vi "FOD.vi"(7 "Yaw":dbl, 8 "DriveMode":enum16{"Meccanum", "Traction"}(ring), 9 "Rotation in":dbl, 10 "Y in":dbl, 11 "X in":dbl) -> (1 "Rotation out":dbl, 2 "Y out":dbl, 3 "X out":dbl)   [LabVIEW 2013]
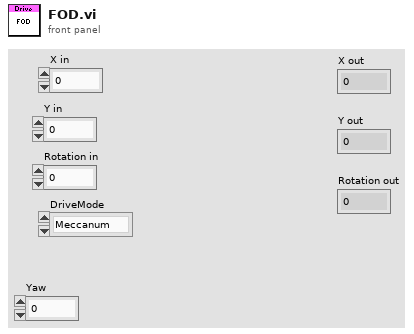
[diagram p1: front panel]
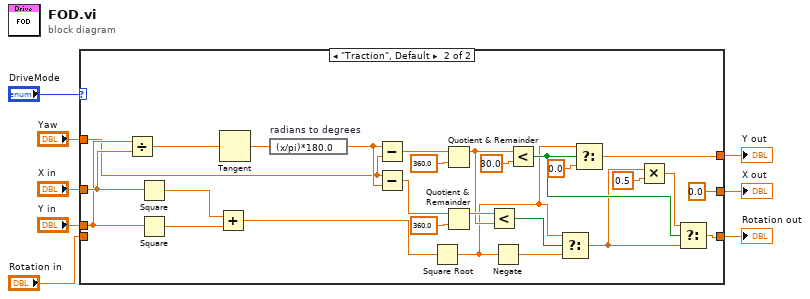
[diagram p0: block diagram]
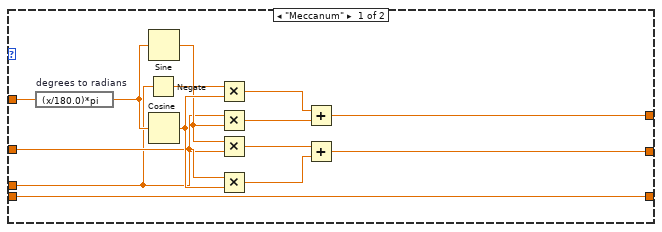
[diagram p2: hidden frame]
diagram:
  n1 = case shown="\"Traction\", Default" "DriveMode" {
    tunnel: [w13 0.0] -> w6
    tunnel: [w14 w38] -> w7
    tunnel: [w12 w35] -> w5
    tunnel: "Rotation in" -> [w12 _]
    tunnel: "X in" -> [w11 w40]
    tunnel: "Y in" -> [w10 w39]
    tunnel: "Yaw" -> [w9 w23]
    frame "Meccanum" {
      n2 = expression code="(x/180.0)*pi" "degrees to radians"(w9) -> (w18:dbl)
      n3 = Negate(x=w10) -> (-x=w15:dbl)
      n4 = Sine(x=w18) -> (sin(x)=w19:dbl)
      n5 = Cosine(x=w18) -> (cos(x)=w20:dbl)
      n6 = Multiply(x=w15, y=w20) -> (x*y=w16:dbl)
      n7 = Multiply(x=w11, y=w19) -> (x*y=w17:dbl)
      n8 = Multiply(x=w19, y=w10) -> (x*y=w21:dbl)
      n9 = Multiply(x=w11, y=w20) -> (x*y=w22:dbl)
      n10 = Add(x=w16, y=w17) -> (x+y=w14:dbl)
      n11 = Add(x=w21, y=w22) -> (x+y=w13:dbl)
    }
    frame "Traction", Default {
      n12 = Divide(x=w39, y=w40) -> (x/y=w49:dbl)
      n13 = Square(x=w40) -> (x^2=w41:dbl)
      n14 = Square(x=w39) -> (x^2=w42:dbl)
      n15 = Add(x=w41, y=w42) -> (x+y=w43:dbl)
      n16 = Tangent(1:w49) -> (0:w48:dbl)
      n17 = expression code="(x/pi)*180.0" "radians to degrees"(w48) -> (w32:dbl)
      n18 = Subtract(x=w32, y=w23) -> (x-y=w46:dbl)
      n19 = Subtract(x=w23, y=w32) -> (x-y=w33:dbl)
      n20 = Square Root(x=w43) -> (sqrt(x)=w24:dbl)
      n21 = Quotient & Remainder(x=w46, y=360.0) -> (x-y*floor(x/y)=w30:dbl)  [unwired: 1 out]
      n22 = Quotient & Remainder(x=w33, y=360.0) -> (x-y*floor(x/y)=w31:dbl)  [unwired: 1 out]
      n23 = Less?(x=w31, y=w30) -> (x < y?=w29:bool)
      n24 = Negate(x=w24) -> (-x=w25:dbl)
      n25 = Less?(x=w30, y=30.0) -> (x < y?=w36:bool)
      n26 = Select(t=w24, s=w29, f=w25) -> (s? t:f=w27:dbl)
      n27 = Select(t=w24, s=w36, f=0.0) -> (s? t:f=w38:dbl)
      n28 = Multiply(x=w27, y=0.5) -> (x*y=w28:dbl)
      n29 = Select(t=w28, s=w36, f=w27) -> (s? t:f=w35:dbl)
    }
  }
  "X out" <- w6
  "Y out" <- w7
  "Rotation out" <- w5
